vi "Cleanup.vi"(8 "error in (no error)":errorcluster, 11 "VMR in":refnum<class "VMR.lvclass">) -> (0 "error out":errorcluster)   [LabVIEW 2022 SP3, in "VMR-Deck.lvlib" / "VMR.lvclass"]
uses:
  VMR.lvclass
  VMR.lvclass/VMR.ctl
  <vilib>/IlluminatedG/IG VoicemeeterRemote API/VoiceMeeterRemote/VoiceMeeterRemote/VoiceMeeterRemote.lvclass
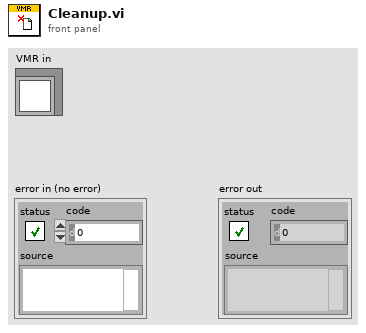
[diagram p1: front panel]
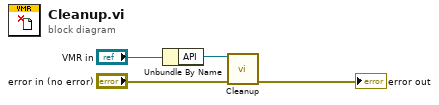
[diagram p0: block diagram]
diagram:
  n1 = Unbundle By Name("VMR in") -> ("API"=w2:refnum<class "VoiceMeeterRemote.lvclass">)
  n2 = call <vilib>:"Cleanup.vi"("error in (no error)"="error in (no error)", "VoiceMeeterRemote in"=w2) -> ("error out"=→"error out":errorcluster)  [unwired: 9 in]
